vi "GE 5565PIORC.Memory.VISA Move Out (DBL).vi"(7 "address space":T1=1 items=["VXI/VME A16"=1, "VXI/VME A24"=2, "VXI/VME A32"=3, "VXI/VME A64"=4, "PXI Memory Allocations"=9, "PXI Configuration"=10, "PXI BAR0"=11, "PXI BAR1"=12, "PXI BAR2"=13, "PXI BAR3"=14, "PXI BAR4"=15, "PXI BAR5"=16], 8 "error in (no error)":errorcluster, 9 "data":dbl[](array[numeric]), 10 "offset (0)":u32, 11 "VISA resource name":refnum<visa-resource-name>) -> (0 "error out":errorcluster, 3 "VISA resource name out":refnum<visa-resource-name>)   [LabVIEW 2016, in "GE 5565PIORC.lvclass"]
uses:
  GE 5565PIORC.lvclass
  <vilib>/Instr/_visa.llb/VISA Register Access Address Space.ctl
  <vilib>/Utility/error.llb/Error Cluster From Error Code.vi
  visa32.dll
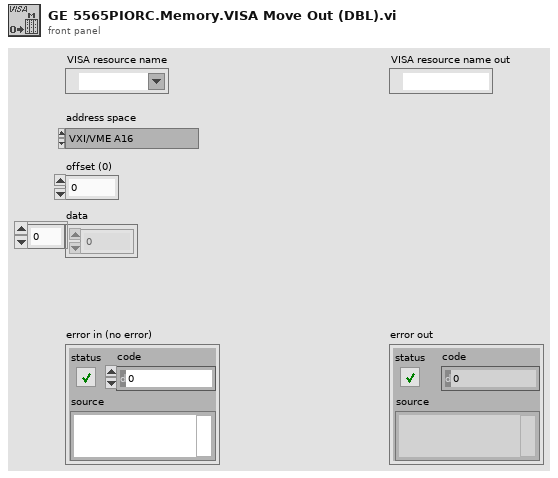
[diagram p1: front panel]
types:
  T1 = typedef "VISA Register Access Address Space.ctl" = u16
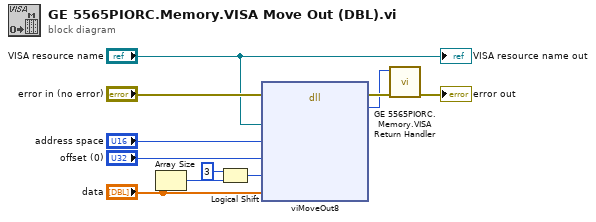
[diagram p0: block diagram]
diagram:
  n1 = Array Size(array="data") -> (size(s)=w7:i32)
  n2 = Logical Shift(y=i16 3, x=w7) -> (x << y=w6:i32)
  n3 = dll-call lib="visa32.*" fn="viMoveOut8"(error in="error in (no error)", "session"="VISA resource name", "address space"="address space", "offset"="offset (0)", "size"=w6, "data"="data") -> (error out=w4:errorcluster, "return type"=w2:i32)  [unwired: 7 in, 1 out]
  n4 = call "GE 5565PIORC.Memory.VISA Return Handler.vi"("error in (no error)"=w4, "VISA return value"=w2) -> ("error out"=→"error out":errorcluster)  [unwired: 9 in]
  "VISA resource name out" <- "VISA resource name"
